vi "test vi.vi"() -> ()   [LabVIEW 2016]
panel:
  in  "JSON String":string="{\n        \"description\": \"the description of the test case\",\n        \"schema\": {\"the schema that should\" : \"be validated against\"},\n        \"tests\": [\n            {\n                \"description\": \"a specific test of a valid instance\",\n                \"data\": \"the instance\",\n                \"valid\": true\n            },\n            {\n                \"description\": \"another specific test this time, invalid\",\n                \"data\": 15,\n                \"valid\": false\n            }\n        ]\n    }"
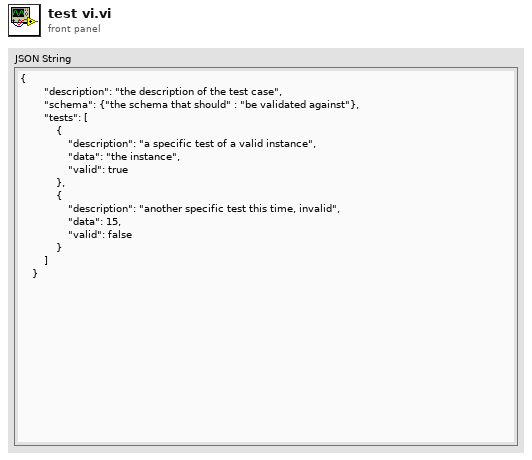
[diagram p1: front panel]
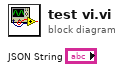
[diagram p0: block diagram]
diagram:
